vi "Reset to factory.vi"(0 "MAC Address in Hex":string) -> (6 "Reset to factory Frame":string)   [LabVIEW 2015]
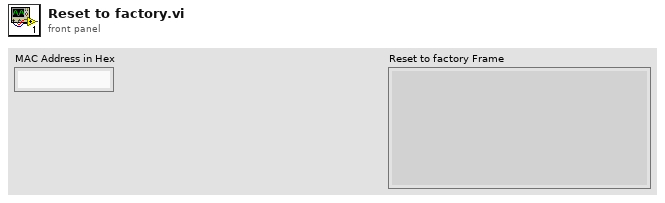
[diagram p1: front panel]
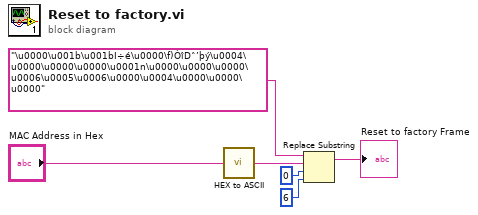
[diagram p0: block diagram]
diagram:
  n1 = call "HEX to ASCII.vi"("String in HEX"="MAC Address in Hex") -> ("String in ASCII"=w5:string)
  n2 = Replace Substring(2:6 ("offset (0)"), 3:0 ("length (len. of substring)"), 4:w5, 5:"\u0000\u001b\u001bI÷é\u0000\f)ÒîDˆ’þý\u0004\u0000\u0000\u0000\u0001n\u0000\u0000\u0000\u0006\u0005\u0006\u0000\u0004\u0000\u0000\u0000") -> (1:→"Reset to factory Frame":string)  [unwired: 1 out]
